vi "Number to Dual.vi"(8 "error in (no error)":errorcluster) -> (0 "error out":errorcluster)   [LabVIEW 2020, in "Tests.lvlib"]
uses:
  Tests.lvlib
  classes/Dual/Dual.lvclass
  6c714974-4a6f-409d-a4f7-6721a31f9ddd.vi
  870bd916-4ec7-440b-a40b-b476b65edc96.vi
  17dd20fb-30ec-44be-99cd-7b04b9e9f501.vi
  29911139-cb8e-4530-803a-9da98143a30b.vi
  dcde96cc-7646-46fa-9b84-6448613c91a3.vi
  870bd916-4ec7-440b-a40b-b476b65edc96.vi/5957e011-cf56-4527-b6ed-13c3a4ca997b.vi
  classes/Dual/Write a.vi
  17dd20fb-30ec-44be-99cd-7b04b9e9f501.vi/5957e011-cf56-4527-b6ed-13c3a4ca997b.vi
  29911139-cb8e-4530-803a-9da98143a30b.vi/5957e011-cf56-4527-b6ed-13c3a4ca997b.vi
  dcde96cc-7646-46fa-9b84-6448613c91a3.vi/5957e011-cf56-4527-b6ed-13c3a4ca997b.vi
  <vilib>/addons/_JKI Toolkits/Caraya/classes/Assert/Assert True.vi
  <vilib>/addons/_JKI Toolkits/Caraya/classes/Test/Test.lvclass
  <vilib>/addons/_JKI Toolkits/Caraya/classes/Assert/Assert.lvclass
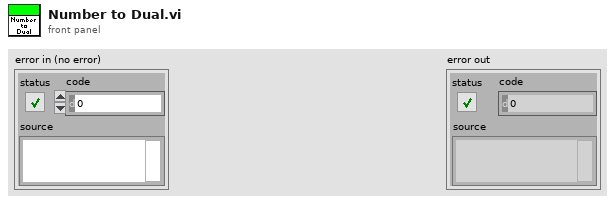
[diagram p1: front panel]
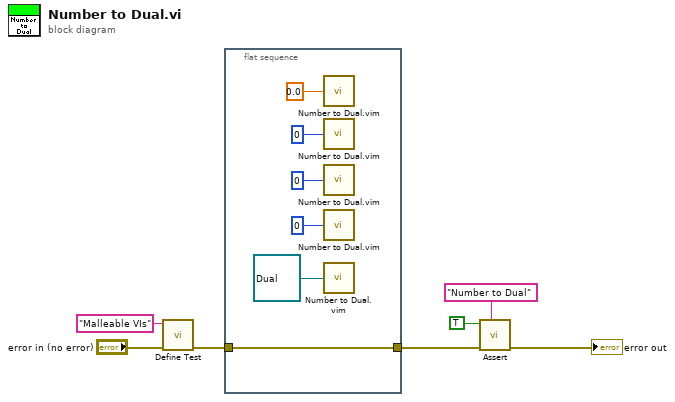
[diagram p0: block diagram]
diagram:
  n1 = call <vilib>:"Define Test.vi"("error in (no error)"="error in (no error)", "Label (VI Title)"="Malleable VIs") -> ("error out"=w3:errorcluster)  [unwired: 9 in]
  n2 = flat-sequence {
    tunnel: w3 -> [w8]
    tunnel: [w8] -> w2
    frame #0 {
      n3 = call "Number to Dual.vim"("Number"=0.0) -> ()  [unwired: 1 out]
      n4 = call "Number to Dual.vim"("Number"=0) -> ()  [unwired: 1 out]
      n5 = call "Number to Dual.vim"("Number"=u32 0) -> ()  [unwired: 1 out]
      n6 = call "Number to Dual.vim"("Number"=u32 0) -> ()  [unwired: 1 out]
      n7 = call "Number to Dual.vim"("Number"=refnum<class "Dual.lvclass"> refnum ("Automatic Differentiation.lvlib:Dual.lvclass")) -> ()  [unwired: 1 out]
    }
  }
  n8 = call-poly <vilib>:"Assert.vi"("Label"="Number to Dual" ("Label (VI Title)"), "error in (no error)"=w2, "True?"=TRUE) -> ("error out"=→"error out":errorcluster)  [unwired: 8 in]
